vi "Starter Kit 2.0 Custom RT Host.vi"() -> ()   [LabVIEW 2013]
doc: "This VI shows how to use hardware abstracted sensor drivers with a custom FPGA VI to control a Starter Kit robot. This VI runs on the RT host. The main FPGA VI must be compiled before this host VI can be run."
uses:
  <vilib>/userdefined/High Color/nirio_resource_hc.ctl
  <instrlib>/DC Motor Controller/HAIOL/DC Motor Controller.lvclass
  <instrlib>/Parallax PING)))/HAIOL/Parallax PING))).lvclass
  <instrlib>/Hitec HS400 Series/HAIOL/Hitec HS400 Series.lvclass
  <vilib>/robotics/Utilities/RPM to Radians per Second (Scalar).vi
  <vilib>/robotics/Utilities/Radians per Second to RPM (Scalar).vi
  <vilib>/rvi/interface/common/niFpgaWaitOnOcc.vi
  <vilib>/FPGAPlugInAG/sbRIO-9632/niLvFpga_Open_sbRIO-9632.vi
  <vilib>/rvi/interface/common/dynamic/niFpgaDynamicAddResources.vi
  <vilib>/Utility/AngleManip/Degrees to Radians (Scalar DBL).vi
  <vilib>/Utility/error.llb/Error Cluster From Error Code.vi
  <vilib>/rvi/errors/niLvFpgaAdjustHostInterfaceError.vi
  <vilib>/FPGAPlugInAG/Dynamic/niLvFpga_Close_Dynamic.vi
  <vilib>/rvi/interface/nirviOpenFPGA/nirviOpenFPGA.xnode
  FPGA Bitfiles/StarterKit2.0FPG_FPGATarget_StarterKit2.0FPG_8D7594C8.lvbitx
  Starter Kit 2.0 Custom FPGA Main.vi
  <vilib>/rvi/interface/nirviReadWriteControl/nirviReadWriteControl.xnode
  <vilib>/rvi/interface/nirviCloseFPGA/nirviCloseFPGA.xnode
  <instrlib>/DC Motor Controller/HAIOL/FPGA/DC Motor Controller FPGA.lvclass
  <instrlib>/Hitec HS400 Series/HAIOL/FPGA/Hitec HS400 Series FPGA.lvclass
  <instrlib>/Parallax PING)))/HAIOL/FPGA/Parallax PING))) FPGA.lvclass
  <vilib>/robotics/Utilities/NI_Robotics Utilities.lvlib
  <vilib>/Utility/AngleManip/NI_AngleManipulation.lvlib
  NiFpgaLv.dll
  <vilib>/rvi/interface/Simulation/niFpgaSimulationCallBeginRW.vi
panel:
  in  "stop":bool
  in  "Left":dbl(slide) min=-100.0 max=100.0 step=4.0 scale=-100.0..100.0
  in  "Right":dbl(slide) min=-100.0 max=100.0 step=4.0 scale=-100.0..100.0
  out "ccw motor velocities":cluster{"Left":dbl, dbl, "Right":dbl, dbl}(graph)
  in  "sensor motor angle":dbl(slide) caption="Sensor Motor Angle (degrees)" scale=90.0..-90.0
  out "PING))) Sensor Distance (m)":dbl(graph)
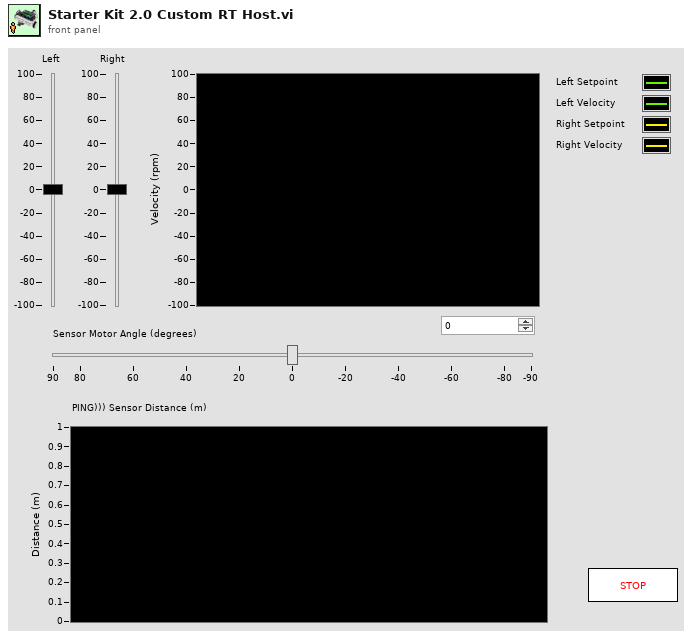
[diagram p1: front panel]
types:
  T1 = typedef "nirio_resource_hc.ctl" = tag
  T2 = cluster{"Left":dbl, "rpm":dbl, "Right":dbl, "rpm":dbl}
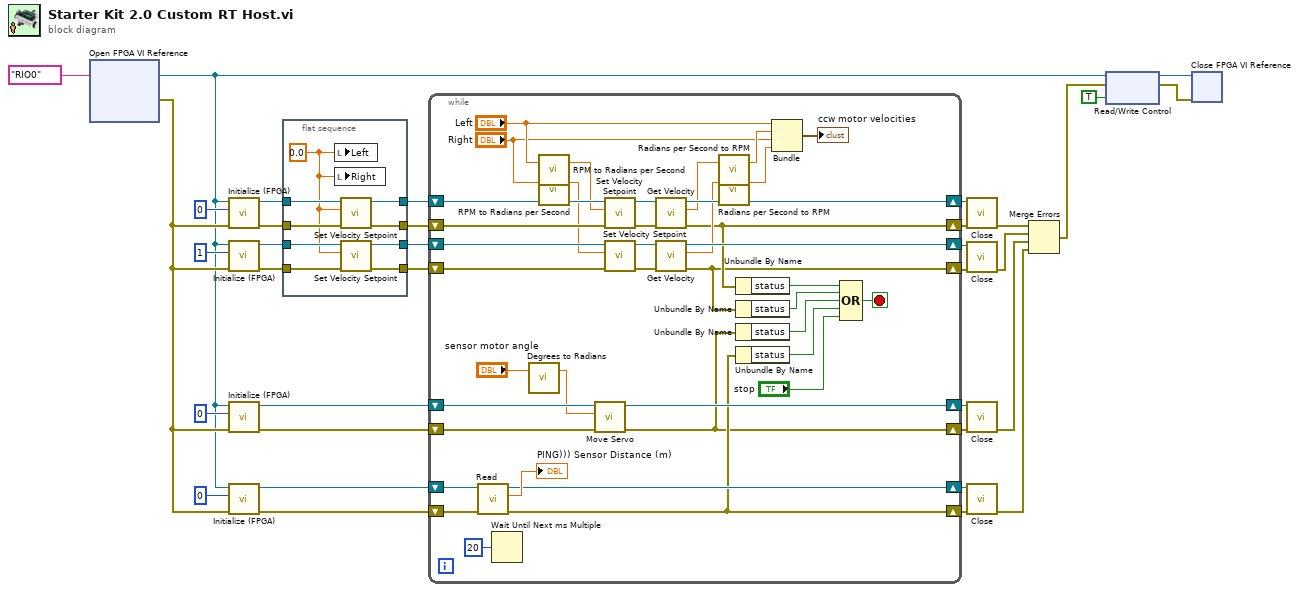
[diagram p0: block diagram]
diagram:
  n1 = xnode "Open FPGA VI Reference"("resource name"=T1 "RIO0") -> ("FPGA VI Reference Out"=w1:refnum<k20>, "error out"=w2:errorcluster)  [unwired: 1 in]
  n2 = call <instrlib>:"Initialize (FPGA).vi"("error in (no error)"=w2, "Actuator ID (0)"=0, "FPGA VI Reference"=w1) -> ("error out"=w9:errorcluster, "DC Motor Controller out"=w11:refnum<class "DC Motor Controller.lvclass">)  [unwired: 7 in]
  n3 = call <instrlib>:"Initialize (FPGA).vi"("error in (no error)"=w2, "Actuator ID (0)"=1, "FPGA VI Reference"=w1) -> ("error out"=w5:errorcluster, "DC Motor Controller out"=w7:refnum<class "DC Motor Controller.lvclass">)  [unwired: 7 in]
  n4 = call <instrlib>:"Initialize (FPGA).vi"("error in (no error)"=w2, "Actuator ID (0)"=0, "FPGA VI Reference"=w1) -> ("error out"=w21:errorcluster, "Hitec HS400 Series out"=w32:refnum<class "Hitec HS400 Series.lvclass">)  [unwired: 7 in]
  n5 = call <instrlib>:"Initialize (FPGA).vi"("error in (no error)"=w2, "Sensor ID (0)"=0, "FPGA VI Reference"=w1) -> ("error out"=w20:errorcluster, "Parallax PING))) out"=w33:refnum<class "Parallax PING))).lvclass">)  [unwired: 7 in]
  n6 = flat-sequence {
    tunnel: w11 -> [w44]
    tunnel: [w43] -> w10
    tunnel: w9 -> [w42]
    tunnel: [w41] -> w8
    tunnel: w7 -> [w40]
    tunnel: [w39] -> w6
    tunnel: w5 -> [w38]
    tunnel: [w37] -> w4
    frame #0 {
      w36 = 0.0 ("CCW Velocity (0 rad/s)")
      n7 = local write "Left"(w36) -> ()
      n8 = local write "Right"(w36) -> ()
      n9 = call-dynamic "Set Velocity Setpoint.vi"("error in (no error)"=w42, "CCW Velocity (0 rad/s)"=w36, "DC Motor Controller in"=w44) -> ("error out"=w41:errorcluster, "DC Motor Controller out"=w43:refnum<class "DC Motor Controller.lvclass">)  [unwired: 7 in]
      n10 = call-dynamic "Set Velocity Setpoint.vi"("error in (no error)"=w38, "CCW Velocity (0 rad/s)"=w36, "DC Motor Controller in"=w40) -> ("error out"=w37:errorcluster, "DC Motor Controller out"=w39:refnum<class "DC Motor Controller.lvclass">)  [unwired: 7 in]
    }
  }
  n11 = while {
    shift-right: [w71] -> w28
    shift-left: w33 -> [w83]
    shift-right: [w68] -> w29
    shift-left: w32 -> [w82]
    shift-right: [w79] -> w31
    shift-left: w10 -> [w81]
    shift-right: [w76] -> w30
    shift-left: w6 -> [w78]
    shift-right: [w61] -> w22
    shift-left: w8 -> [w75]
    shift-right: [w60] -> w17
    shift-left: w4 -> [w67]
    shift-right: [w58] -> w19
    shift-left: w21 -> [w69]
    shift-right: [w59] -> w18
    shift-left: w20 -> [w70]
    stop <- w52 stop-if-true
    n12 = call-dynamic "Read.vi"("error in (no error)"=w70, "Parallax PING))) in"=w83) -> ("error out"=w59:errorcluster, "Distance (m)"=→"PING))) Sensor Distance (m)":dbl, "Parallax PING))) out"=w71:refnum<class "Parallax PING))).lvclass">)  [unwired: 6 in, 1 out]
    n13 = Wait Until Next ms Multiple(millisecond multiple=u32 20) -> ()  [unwired: 1 out]
    n14 = call-poly <vilib>:"Degrees to Radians.vi"("angle (deg)"="sensor motor angle") -> ("angle (rad)"=w45:dbl)  [unwired: 2 in]
    n15 = call-poly <vilib>:"RPM to Radians per Second.vi"("rpm"="Left") -> ("radians per second"=w62:dbl)  [unwired: 2 in]
    n16 = call-poly <vilib>:"RPM to Radians per Second.vi"("rpm"="Right") -> ("radians per second"=w63:dbl)  [unwired: 2 in]
    n17 = call-dynamic "Move Servo.vi"("error in (no error)"=w69, "CCW Position (0.0 rad)"=w45, "Hitec HS400 Series in"=w82) -> ("error out"=w58:errorcluster, "Hitec HS400 Series out"=w68:refnum<class "Hitec HS400 Series.lvclass">)  [unwired: 7 in]
    n18 = call-dynamic "Set Velocity Setpoint.vi"("error in (no error)"=w75, "CCW Velocity (0 rad/s)"=w62, "DC Motor Controller in"=w81) -> ("error out"=w74:errorcluster, "DC Motor Controller out"=w80:refnum<class "DC Motor Controller.lvclass">)  [unwired: 7 in]
    n19 = call-dynamic "Set Velocity Setpoint.vi"("error in (no error)"=w67, "CCW Velocity (0 rad/s)"=w63, "DC Motor Controller in"=w78) -> ("error out"=w66:errorcluster, "DC Motor Controller out"=w77:refnum<class "DC Motor Controller.lvclass">)  [unwired: 7 in]
    n20 = call-dynamic "Get Velocity.vi"("error in (no error)"=w74, "DC Motor Controller in"=w80) -> ("error out"=w61:errorcluster, "CCW Velocity (rad/s)"=w65:dbl, "DC Motor Controller out"=w79:refnum<class "DC Motor Controller.lvclass">)  [unwired: 7 in]
    n21 = call-dynamic "Get Velocity.vi"("error in (no error)"=w66, "DC Motor Controller in"=w77) -> ("error out"=w60:errorcluster, "CCW Velocity (rad/s)"=w64:dbl, "DC Motor Controller out"=w76:refnum<class "DC Motor Controller.lvclass">)  [unwired: 7 in]
    n22 = call-poly <vilib>:"Radians per Second to RPM.vi"("radians per second"=w65) -> ("rpm"=w50:dbl)  [unwired: 2 in]
    n23 = call-poly <vilib>:"Radians per Second to RPM.vi"("radians per second"=w64) -> ("rpm"=w48:dbl)  [unwired: 2 in]
    n24 = Unbundle By Name(w61) -> ("status"=w57:bool)
    n25 = Unbundle By Name(w60) -> ("status"=w56:bool)
    n26 = Unbundle By Name(w58) -> ("status"=w55:bool)
    n27 = Unbundle By Name(w59) -> ("status"=w54:bool)
    n28 = Bundle("Left"="Left", "rpm"=w50, "Right"="Right", "rpm"=w48) -> (→"ccw motor velocities":T2)  [unwired: 1 in]
    n29 = Compound Arithmetic op=OR(w57, w56, w55, w54, "stop") -> (w52:bool)
  }
  n30 = call-dynamic "Close.vi"("error in (no error)"=w22, "DC Motor Controller in"=w31) -> ("error out"=w16:errorcluster)  [unwired: 9 in]
  n31 = call-dynamic "Close.vi"("error in (no error)"=w17, "DC Motor Controller in"=w30) -> ("error out"=w15:errorcluster)  [unwired: 9 in]
  n32 = call-dynamic "Close.vi"("error in (no error)"=w19, "Hitec HS400 Series in"=w29) -> ("error out"=w14:errorcluster)  [unwired: 9 in]
  n33 = call-dynamic "Close.vi"("error in (no error)"=w18, "Parallax PING))) in"=w28) -> ("error out"=w13:errorcluster)  [unwired: 9 in]
  n34 = Merge Errors(w16, w15, w14, w13) -> (w12:errorcluster)
  n35 = xnode "Read/Write Control"("FPGA VI Reference In"=w1, "error in"=w12, "stop"=TRUE) -> ("FPGA VI Reference Out"=w25:refnum<k20>, "error out"=w24:errorcluster)
  n36 = xnode "Close FPGA VI Reference"("FPGA VI Reference In"=w25, "error in"=w24) -> ()  [unwired: 1 out]
